vi "数据写入临时表格.vi"(6 "组合框":string(combo), 7 "表格选择":string(combo)="database1.mdb", 8 "error in":errorcluster caption="error out", 9 "存储表格":string(combo)="databasetp1.mdb", 10 "table":string, 11 "data":string[][](table)) -> (0 "error out":errorcluster)   [LabVIEW 2016]
uses:
  <vilib>/Utility/sysdir.llb/System Directory Type.ctl
  <vilib>/addons/database/Connection.llb/DB Tools Open Connec (String).vi
  <vilib>/addons/database/NI_Database_API.lvlib
panel:
  out "簇":T1 {"时间标识" format="%<%Y/%m/%d %H:%M:%S>T"}
  in  "columns":string[](array[string])=["时间", "测量模式", "数据类型", "检测值", "单位", "数据标识", "因子编码", "标样参考值", "F0", "F1", "F2", "F3", "温度", "湿度", "量程标识", "SN"]
  # "databasetp.mdb"
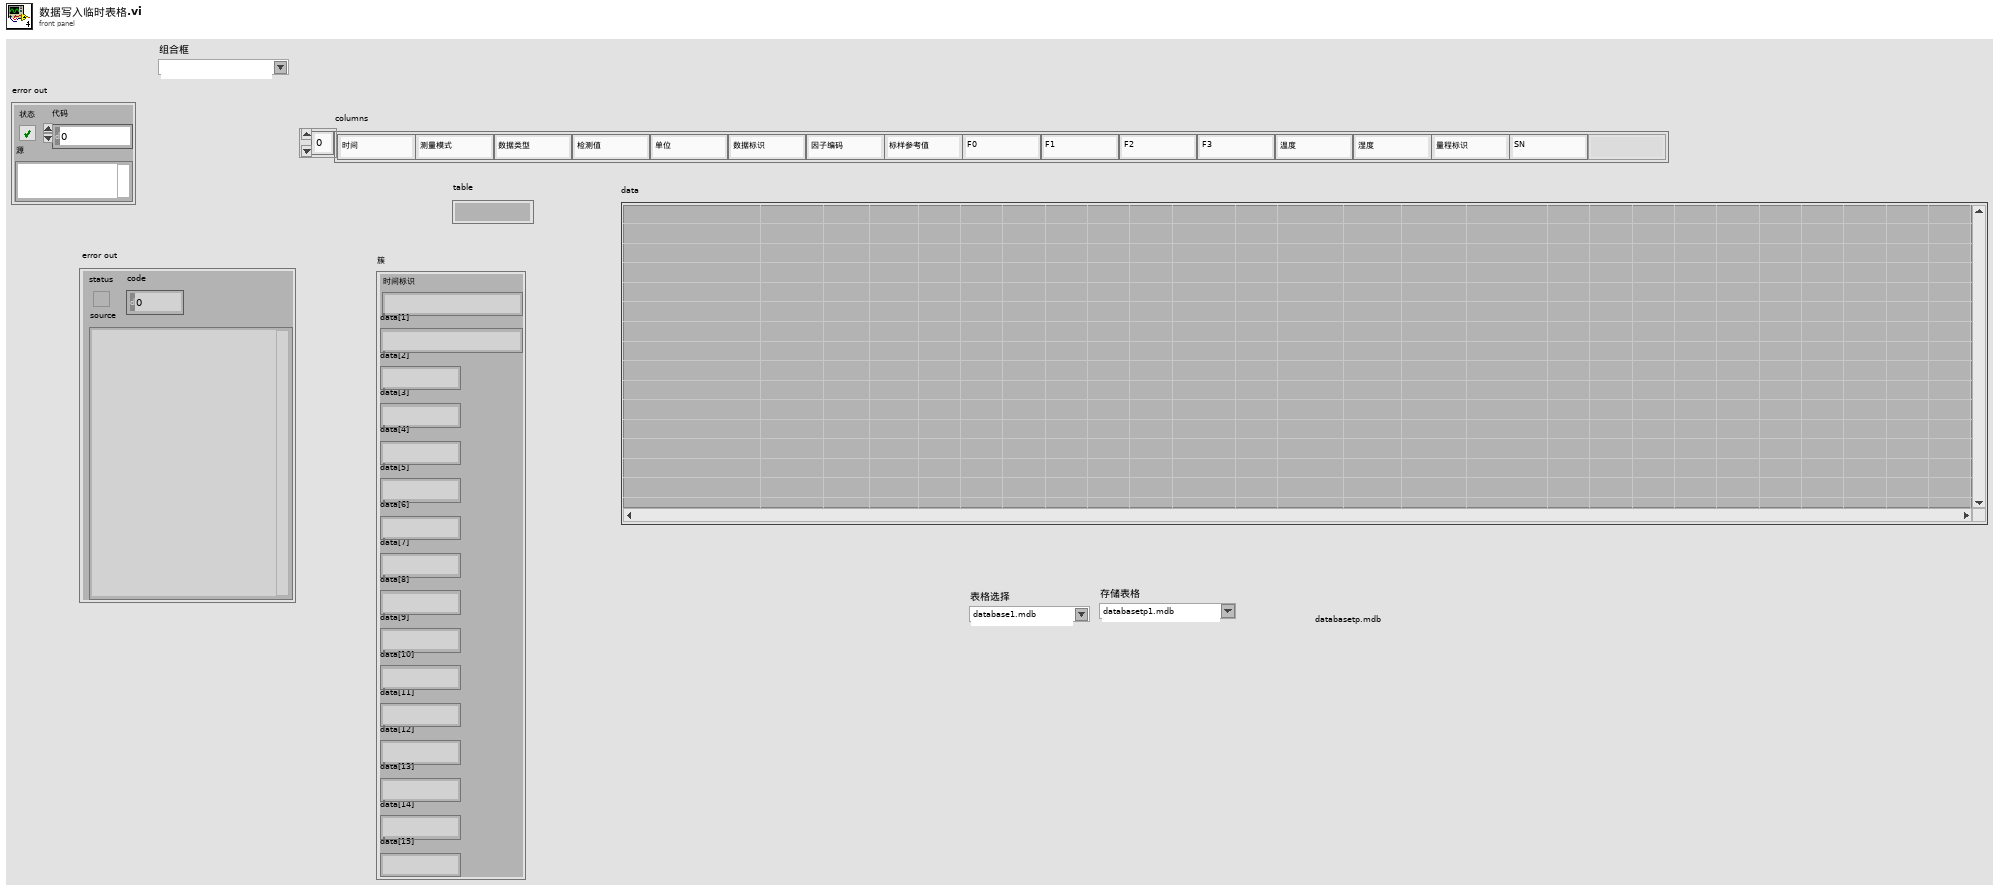
[diagram p1: front panel]
types:
  T1 = cluster{"时间标识":timestamp, "data[1]":string, "data[2]":string, "data[3]":string, "data[4]":string, "data[5]":string, "data[6]":string, "data[7]":string, "data[8]":string, "data[9]":string, "data[10]":string, "data[11]":string, "data[12]":string, "data[13]":string, "data[14]":string, "data[15]":string}
  T2 = typedef "System Directory Type.ctl" = i32
  T3 = cluster{"data[0]":string, "data[1]":string, "data[2]":string, "data[3]":string, "data[4]":string, "data[5]":string, "data[6]":string, "data[7]":string, "data[8]":string, "data[9]":string, "data[10]":string, "data[11]":string, "data[12]":string, "data[13]":string, "data[14]":string, "data[15]":string}
  T4 = typedef "NI_Database_API.lvlib/Conn ObjectReference.ctl" = refnum<k1>
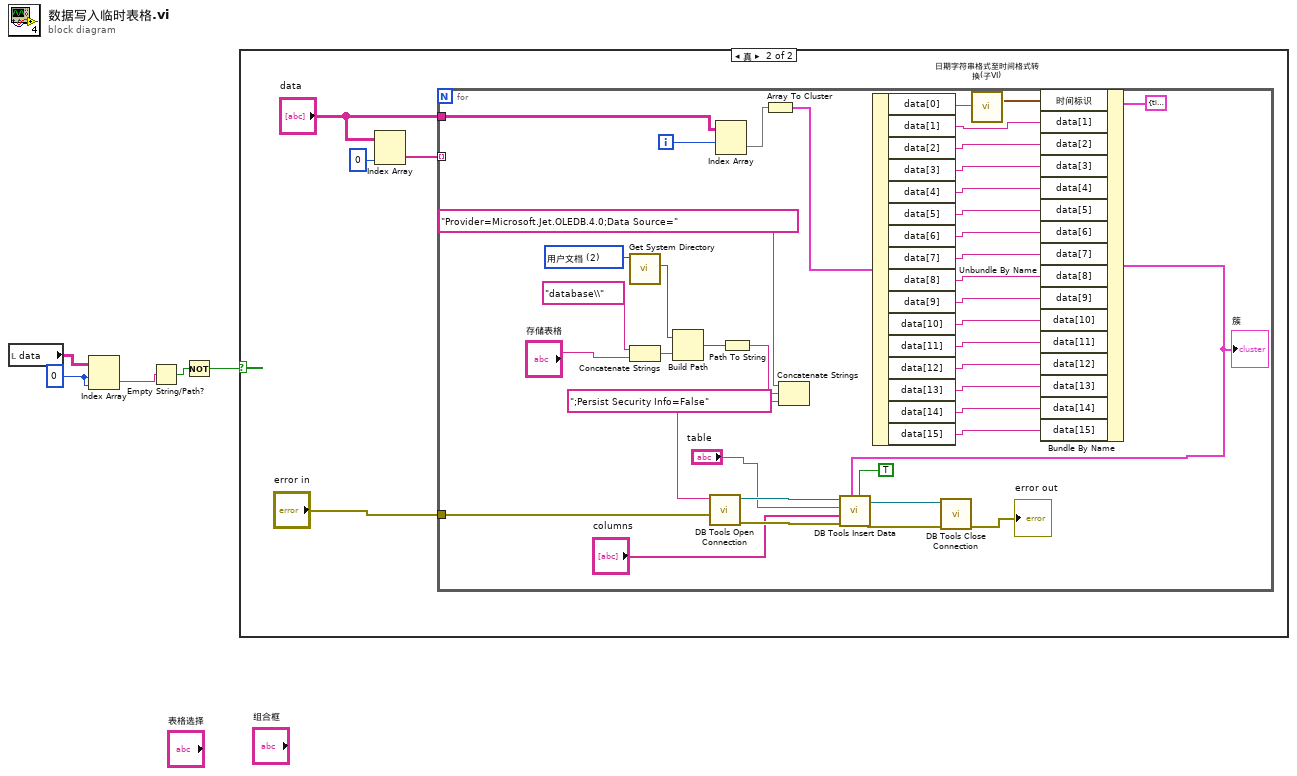
[diagram p0: block diagram]
diagram:
  w4 = 0 ("索引 (行)")
  n1 = local read "data"() -> (w5:string[][])
  n2 = Index Array(array=w5, index (row)=w4, index (col)=w4) -> (element=w3:string)
  n3 = Empty String/Path?(string/path=w3) -> (empty?=w2:bool)
  n4 = Not(x=w2) -> (.not. x?=w1:bool)
  n5 = case shown="真" w1 {
    frame False {
    }
    frame True {
      n6 = Index Array(array="data", index (col)=0 ("禁用的索引 (列)")) -> (element=w7:string[])  [unwired: 1 in]
      n7 = for {
        tunnel: "error in" -> [w51]
        tunnel: "data" -> [w13]
        tunnel: w7 -> [_] mode=indexing
        i -> [w12]
        w43 = T2 2 items=["用户目录"=0, "用户桌面"=1, "用户文档"=2, "用户应用程序数据"=3, "用户设置"=4, "用户临时目录"=5, "公共文档"=6, "公共应用程序数据"=7, "公共设置"=8, "公共缓存"=13, "系统核心库"=9, "系统安装库"=10, "应用程序文件"=11, "启动盘根目录"=12] ("system directory type")
        n8 = call <vilib>:"Get System Directory.vi"("system directory type"=w43) -> ("system directory"=w45:path)  [unwired: 10 in]
        n9 = Concatenate Strings("database\\" ("condition"), "存储表格") -> (w50:string)
        n10 = Build Path(base path=w45, name or relative path=w50) -> (appended path=w46:path)
        n11 = Index Array(array=w13, index (row)=w12) -> (element=w35:string[])  [unwired: 1 in]
        n12 = Path To String(path=w46) -> (string=w47:string)
        n13 = Array To Cluster(array=w35) -> (cluster=w34:T3)
        n14 = Concatenate Strings("Provider=Microsoft.Jet.OLEDB.4.0;Data Source=" ("condition"), w47, ";Persist Security Info=False" ("condition")) -> (w42:string)
        n15 = call-poly <vilib>:"DB Tools Open Connection.vi"("error in (no error)"=w51, "connection information"=w42) -> ("error out"=w40:errorcluster, "connection reference"=w41:T4)  [unwired: 6 in]
        n16 = Unbundle By Name(w34) -> ("data[0]"=w33:string, "data[1]"=w28:string, "data[2]"=w27:string, "data[3]"=w26:string, "data[4]"=w25:string, "data[5]"=w24:string, "data[6]"=w23:string, "data[7]"=w22:string, "data[8]"=w21:string, "data[9]"=w20:string, "data[10]"=w19:string, "data[11]"=w18:string, "data[12]"=w17:string, "data[13]"=w16:string, "data[14]"=w15:string, "data[15]"=w14:string)
        n17 = call "日期字符串格式至时间格式转换(子VI).vi"("data[0]"=w33) -> ("time stamp"=w31:timestamp)  [unwired: 10 in]
        n18 = Bundle By Name(cluster=T1 {"时间标识"=timestamp(0 s since 1904-01-01), "data[1]"="水样测试", "data[2]"="N", "data[3]"="6.67", "data[4]"="mg/L", "data[5]"="T\u0000\u0000\u0000\u0000\u0000\u0000\u0000\u0000\u0000\u0000\u0000", "data[6]"="w21003", "data[7]"="0", "data[8]"="3282", "data[9]"="621", "data[10]"=".723047", "data[11]"="0", "data[12]"="22.88086", "data[13]"="55.39742", "data[14]"="92-1-1", "data[15]"="70G18G022\u0000\u0000\u0000"} ("簇"), "时间标识"=w31, "data[1]"=w28, "data[2]"=w27, "data[3]"=w26, "data[4]"=w25, "data[5]"=w24, "data[6]"=w23, "data[7]"=w22, "data[8]"=w21, "data[9]"=w20, "data[10]"=w19, "data[11]"=w18, "data[12]"=w17, "data[13]"=w16, "data[14]"=w15, "data[15]"=w14) -> (w30:T1)
        "簇" <- w30
        n19 = call <vilib>:"DB Tools Insert Data.vi"("create table? (F)"=TRUE, "data"=w30, "error in (no error)"=w40, "columns"="columns", "table"="table", "connection reference"=w41) -> ("error out"=w37:errorcluster, "connection reference out"=w38:T4)  [unwired: 4 in]
        n20 = call <vilib>:"DB Tools Close Connection.vi"("error in (no error)"=w37, "connection reference"=w38) -> ("error out"=→"error out":errorcluster)  [unwired: 5 in]
      }
    }
  }
